vi "TxtFile Load.vi"(8 "error in (no error)":errorcluster, 11 "Path":path) -> (0 "error out":errorcluster, 3 "text":string)   [LabVIEW 2012]
doc: "Use this template to build a VI to use as a subVI."
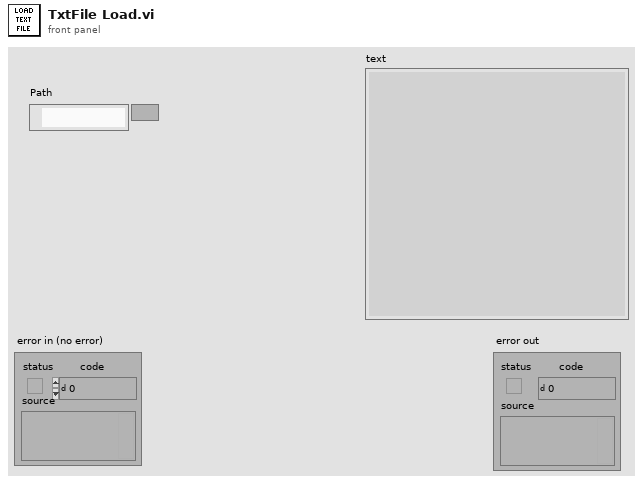
[diagram p1: front panel]
types:
  T1 = enum16{"open", "replace", "create", "open or create", "replace or create", "replace or create with confirmation"}
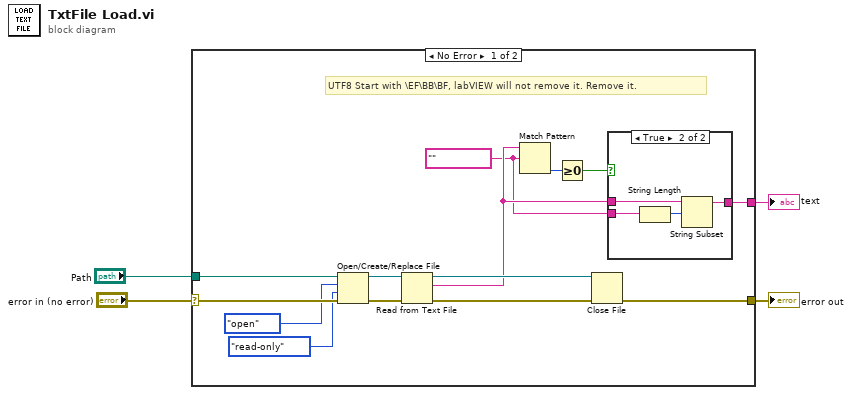
[diagram p0: block diagram]
diagram:
  n1 = case shown="No Error" "error in (no error)" {
    selector: "error in (no error)" -> [w18 w24]
    tunnel: [w10 w24] -> w3
    tunnel: "Path" -> [w17 _]
    tunnel: [w7 _] -> w1
    frame No Error {
      w5 = "﻿" ("regular expression")
      # "UTF8 Start with \\EF\\BB\\BF, labVIEW will not remove it. Remove it."
      n2 = Open/Create/Replace File(file path (use dialog)=w17, error in=w18, operation (0:open)=T1."open", access (0:read/write)=enum16{"read/write", "read-only", "write-only"}."read-only") -> (refnum out=w14:refnum<file>, error out=w11:errorcluster)  [unwired: 2 in, 1 out]
      n3 = Read from Text File(file (use dialog)=w14, error in=w11) -> (refnum out=w13:refnum<file>, text=w8:string, error out=w12:errorcluster)  [unwired: 2 in, 1 out]
      n4 = Match Pattern(string=w8, regular expression=w5) -> (offset past match=w9:i32)  [unwired: 1 in, 3 out]
      n5 = Greater Or Equal To 0?(x=w9) -> (x >= 0?=w6:bool)
      n6 = Close File(refnum=w13, error in=w12) -> (error out=w10:errorcluster)  [unwired: 1 out]
      n7 = case shown="True" w6 {
        tunnel: w8 -> [w19 w23]
        tunnel: [w19 w22] -> w7
        tunnel: w5 -> [_ w20]
        frame False {
        }
        frame True {
          n8 = String Length(string=w20) -> (length=w21:i32)
          n9 = String Subset(string=w23, offset (0)=w21) -> (substring=w22:string)  [unwired: 1 in]
        }
      }
    }
    frame Error {
    }
  }
  "error out" <- w3
  "text" <- w1
